vi "复杂反馈节点.vi"() -> ()   [LabVIEW 2020]
panel:
  out "result":dbl
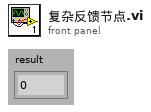
[diagram p1: front panel]
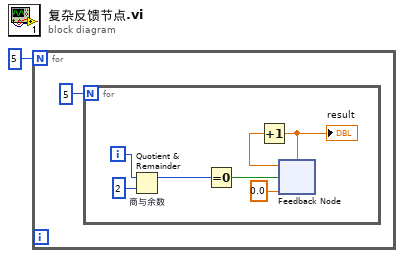
[diagram p0: block diagram]
diagram:
  n1 = for {
    N: 5 -> [_]
    n2 = for {
      N: 5 -> [_]
      i -> [w3]
      n3 = Quotient & Remainder "商与余数"(x=w3, y=2) -> (x-y*floor(x/y)=w5:i32)  [unwired: 1 out]
      n4 = Equal To 0?(x=w5) -> (x = 0?=w4:bool)
      n5 = feedback #1(0.0) -> (w8:dbl)
      n6 = Increment(x=w8) -> (x+1=w9:dbl)
      "result" <- w9
      n7 = feedback-in #1(w9, w4) -> ()
    }
  }
